vi "Write B_msg Msg.vi"(10 "B_Actor.lvlib:B_msg Msg.lvclass":refnum<class "B_msg Msg.lvclass">, 11 "B_Actor in":refnum<class "B_Actor.lvclass">) -> (3 "B_Actor out":refnum<class "B_Actor.lvclass">)   [LabVIEW 2025, in "B_Actor.lvlib" / "B_Actor.lvclass"]
uses:
  B_Actor.lvclass
  B_Actor Messages/B_msg Msg/B_msg Msg.lvclass
  B_Actor.lvclass/B_Actor.ctl
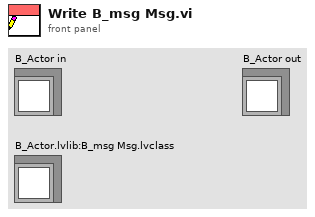
[diagram p1: front panel]
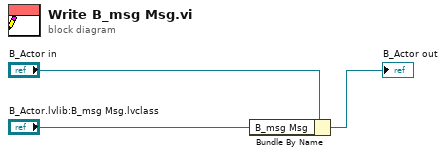
[diagram p0: block diagram]
diagram:
  n1 = Bundle By Name(cluster="B_Actor in", "B_msg Msg"="B_Actor.lvlib:B_msg Msg.lvclass") -> (→"B_Actor out":refnum<class "B_Actor.lvclass">)
